vi "Check Needs HTTPS.vi"(8 "error in (no error)":errorcluster, 11 "Processing In":refnum<class "Processing.lvclass">) -> (0 "error out":errorcluster, 2 "HTTPS Upgrade?":bool, 3 "Processing out":refnum<class "Processing.lvclass">)   [LabVIEW 2020, in "HTTP Server.lvlib" / "Server.lvclass"]
uses:
  Server.lvclass
  Processing/Processing.lvclass
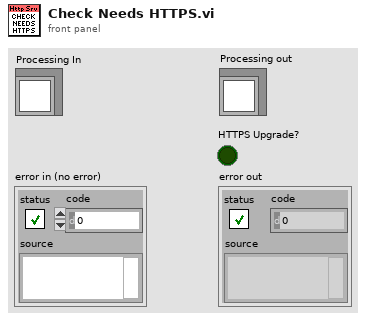
[diagram p1: front panel]
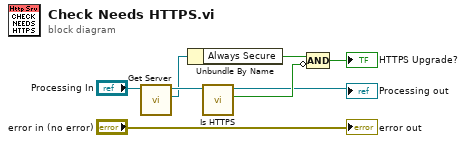
[diagram p0: block diagram]
diagram:
  n1 = call "Get Server.vi"("Processing in"="Processing In") -> ("Server"=w1:refnum<class "Server.lvclass">, "Processing out"=w2:refnum<class "Processing.lvclass">)  [unwired: 9 in]
  n2 = Unbundle By Name(w1) -> ("Always Secure"=w6:bool)
  n3 = call "Is HTTPS.vi"("Processing in"=w2) -> ("HTTPS?"=w7:bool, "Processing out"=→"Processing out":refnum<class "Processing.lvclass">)  [unwired: 8 in, 1 out]
  n4 = Compound Arithmetic op=AND(w6, invert w7) -> (→"HTTPS Upgrade?":bool)
  "error out" <- "error in (no error)"
